vi "Read Server Files.vi"(6 "Error Message in":string, 8 "Error In":errorcluster) -> (0 "Error Out":errorcluster, 3 "Server Files Cluster":T1, 4 "Error Message out":string)   [LabVIEW 2019]
uses:
  <vilib>/Utility/config.llb/Read Key (String).vi
  <vilib>/Utility/config.llb/Write Key (String).vi
  <vilib>/Utility/config.llb/NI_LVConfig.lvlib
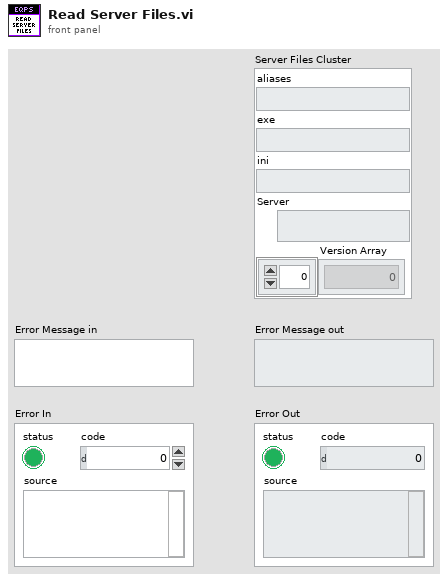
[diagram p1: front panel]
types:
  T1 = cluster{"aliases":string, "exe":string, "ini":string, "Server":path, "Version Array":i32[]}
  T2 = typedef "NI_LVConfig.lvlib/Config Data RefNum.ctl" = refnum<k1>
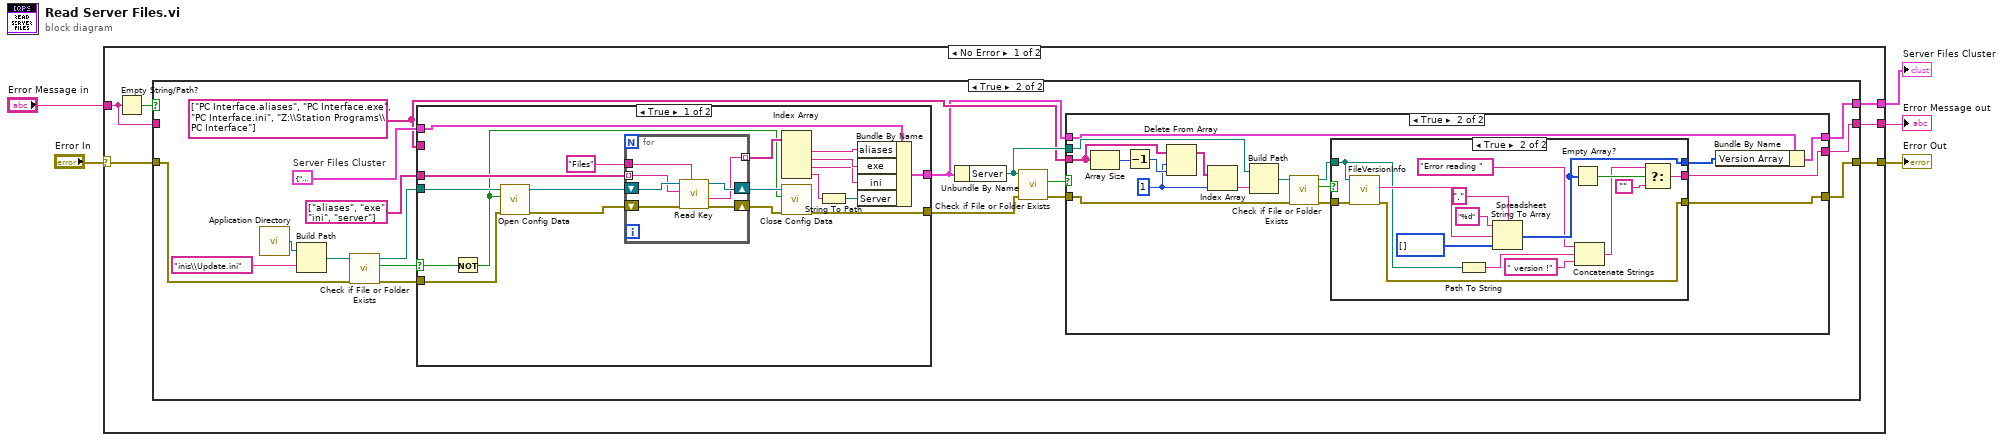
[diagram p0: block diagram]
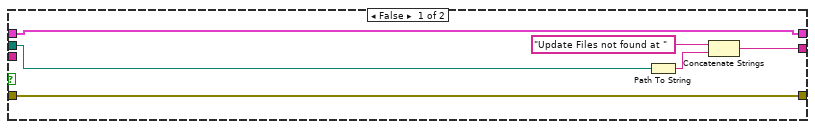
[diagram p3: hidden frame]
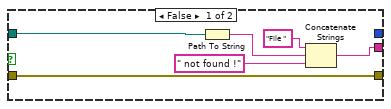
[diagram p4: hidden frame]
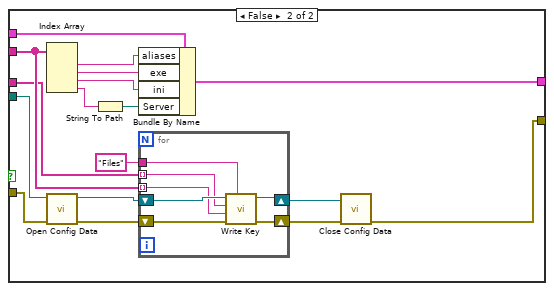
[diagram p5: hidden frame]
diagram:
  n1 = case shown="No Error" "Error In" {
    selector: "Error In" -> [w7 w127]
    tunnel: [w8 w127] -> w4
    tunnel: [w10 w126] -> w3
    tunnel: "Error Message in" -> [w9 w126]
    tunnel: [w6 _] -> w1
    frame No Error {
      n2 = Empty String/Path?(string/path=w9) -> (empty?=w11:bool)
      n3 = case shown="True" w11 {
        tunnel: [w13 w18] -> w10
        tunnel: w9 -> [w13 _]
        tunnel: [w12 w17] -> w8
        tunnel: w7 -> [w12 w25]
        tunnel: [_ w14] -> w6
        frame False {
        }
        frame True {
          w24 = T1 {"aliases"="", "exe"="", "ini"="", "Server"=path "", "Version Array"=[]}  # Server Files Cluster
          w16 = string[] ["PC Interface.aliases", "PC Interface.exe", "PC Interface.ini", "Z:\\Station Programs\\PC Interface"]
          n4 = call <vilib>:"Application Directory.vi"() -> ("Application Directory"=w31:path)
          n5 = Build Path(base path=w31, name or relative path="inis\\Update.ini") -> (appended path=w29:path)
          n6 = call <vilib>:"Check if File or Folder Exists.vi"("error in (no error)"=w25, "path"=w29) -> ("error out"=w28:errorcluster, "file or folder exists?"=w27:bool, "dup path"=w26:path)  [unwired: 7 in]
          n7 = case shown="True" w27 {
            selector: w27 -> [w78 _]
            tunnel: w28 -> [w94 w118]
            tunnel: w26 -> [w93 w117]
            tunnel: [w90 w114] -> w22
            tunnel: w16 -> [_ w105]
            tunnel: [w76 w104] -> w15
            tunnel: w24 -> [w80 w103]
            tunnel: string[] ["aliases", "exe", "ini", "server"] -> [w79 w102]
            frame True {
              n8 = Not(x=w78) -> (.not. x?=w77:bool)
              n9 = call <vilib>:"Open Config Data.vi"("error in (no error)"=w94, "create file if necessary (T)"=w77, "configuration file path"=w93) -> ("error out"=w92:errorcluster, "refnum"=w91:T2)  [unwired: 6 in, 1 out]
              n10 = for {
                tunnel: "Files" -> [w99]
                shift-right: [w97] -> w87
                shift-left: w92 -> [w101]
                shift-right: [w98] -> w88
                shift-left: w91 -> [w100]
                tunnel: w79 -> [w96] mode=indexing
                tunnel: [w95] -> w86 mode=indexing
                n11 = call-poly <vilib>:"Read Key.vi"("section"=w99, "error in (no error)"=w101, "key"=w96, "refnum"=w100) -> ("error out"=w97:errorcluster, "value"=w95:string, "refnum out"=w98:T2)  [unwired: 4 in, 1 out]
              }
              n12 = Index Array(array=w86) -> (element #1=w85:string, element #2=w84:string, element #3=w83:string, element #4=w82:string)  [unwired: 4 in]
              n13 = call <vilib>:"Close Config Data.vi"("error in (no error)"=w87, "write file if changed (T)"=w77, "refnum"=w88) -> ("error out"=w90:errorcluster)  [unwired: 7 in, 1 out]
              n14 = String To Path(string=w82) -> (path=w81:path)
              n15 = Bundle By Name(cluster=w80, "aliases"=w85, "exe"=w84, "ini"=w83, "Server"=w81) -> (w76:T1)
            }
            frame False {
              n16 = Index Array(array=w105) -> (element #1=w110:string, element #2=w109:string, element #3=w108:string, element #4=w107:string)  [unwired: 4 in]
              n17 = call <vilib>:"Open Config Data.vi"("error in (no error)"=w118, "configuration file path"=w117) -> ("error out"=w116:errorcluster, "refnum"=w115:T2)  [unwired: 7 in, 1 out]
              n18 = String To Path(string=w107) -> (path=w106:path)
              n19 = Bundle By Name(cluster=w103, "aliases"=w110, "exe"=w109, "ini"=w108, "Server"=w106) -> (w104:T1)
              n20 = for {
                tunnel: "Files" -> [w123]
                shift-right: [w121] -> w111
                shift-left: w116 -> [w125]
                shift-right: [w122] -> w112
                shift-left: w115 -> [w124]
                tunnel: w102 -> [w120] mode=indexing
                tunnel: w105 -> [w119] mode=indexing
                n21 = call-poly <vilib>:"Write Key.vi"("section"=w123, "error in (no error)"=w125, "value"=w119, "key"=w120, "refnum"=w124) -> ("error out"=w121:errorcluster, "refnum out"=w122:T2)  [unwired: 4 in, 1 out]
              }
              n22 = call <vilib>:"Close Config Data.vi"("error in (no error)"=w111, "refnum"=w112) -> ("error out"=w114:errorcluster)  [unwired: 8 in, 1 out]
            }
          }
          n23 = Unbundle By Name(w15) -> ("Server"=w19:path)
          n24 = call <vilib>:"Check if File or Folder Exists.vi"("error in (no error)"=w22, "path"=w19) -> ("error out"=w21:errorcluster, "file or folder exists?"=w20:bool)  [unwired: 7 in, 1 out]
          n25 = case shown="True" w20 {
            tunnel: w21 -> [w33 w50]
            tunnel: w19 -> [w37 w51]
            tunnel: [w34 w41] -> w18
            tunnel: [w33 w49] -> w17
            tunnel: w16 -> [_ w53]
            tunnel: w15 -> [w32 w40]
            tunnel: [w32 w38] -> w14
            frame False {
              n26 = Path To String(path=w37) -> (string=w35:string)
              n27 = Concatenate Strings("Update Files not found at ", w35) -> (w34:string)
            }
            frame True {
              w43 = 1 ("length")
              n28 = Array Size(array=w53) -> (size(s)=w54:i32)
              n29 = Decrement(x=w54) -> (x-1=w52:i32)
              n30 = Delete From Array(array=w53, length=w43, index=w52) -> (array with subset deleted=w44:string[])  [unwired: 1 out]
              n31 = Index Array(array=w44, index=w43) -> (element=w42:string)
              n32 = Build Path(base path=w51, name or relative path=w42) -> (appended path=w48:path)
              n33 = call <vilib>:"Check if File or Folder Exists.vi"("error in (no error)"=w50, "path"=w48) -> ("error out"=w47:errorcluster, "file or folder exists?"=w46:bool, "dup path"=w45:path)  [unwired: 7 in]
              n34 = case shown="True" w46 {
                tunnel: w47 -> [w60 w75]
                tunnel: w45 -> [w57 w67]
                tunnel: [w60 w73] -> w49
                tunnel: [_ w69] -> w39
                tunnel: [w55 w62] -> w41
                frame False {
                  n35 = Path To String(path=w57) -> (string=w56:string)
                  n36 = Concatenate Strings("File ", w56, " not found !") -> (w55:string)
                }
                frame True {
                  n37 = call <vilib>:"FileVersionInfo.vi"("error in (no error)"=w75, "Application Path in"=w67) -> ("error out"=w73:errorcluster, "File Version Info"=w74:string)  [unwired: 6 in, 2 out]
                  n38 = Path To String(path=w67) -> (string=w65:string)
                  n39 = Spreadsheet String To Array(delimiter (Tab)=".", format string="%d", spreadsheet string=w74, array type (2D Dbl)=i32[] []) -> (array=w69:i32[])
                  n40 = Empty Array?(array=w69) -> (empty?=w68:bool)
                  n41 = Concatenate Strings("Error reading ", w65, " version !") -> (w63:string)
                  n42 = Select(t=w63, s=w68, f="") -> (s? t:f=w62:string)
                }
              }
              n43 = Bundle By Name(cluster=w40, "Version Array"=w39) -> (w38:T1)
            }
          }
        }
      }
    }
    frame Error {
    }
  }
  "Error Out" <- w4
  "Error Message out" <- w3
  "Server Files Cluster" <- w1
